vi "DequeueDependency.vi"(8 "error in (no error)":errorcluster, 11 "CDependencyQueue in":refnum<class "CDependencyQueue.lvclass">) -> (0 "error out":errorcluster, 1 "Shallow deps?":bool, 2 "Path":path, 3 "CDependencyQueue out":refnum<class "CDependencyQueue.lvclass">, 5 "timed out?":bool)   [LabVIEW 2020, in "DependencyInspection.lvlib" / "CDependencyQueue.lvclass"]
uses:
  CDependencyQueue.lvclass
  CDependencyQueue.lvclass/CDependencyQueue.ctl
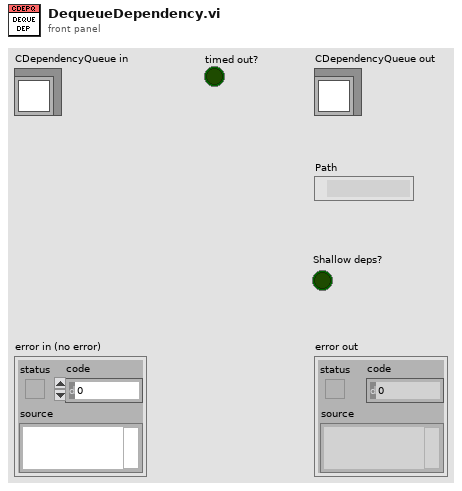
[diagram p1: front panel]
types:
  T1 = typedef "DependencyInspection.lvlib/CDependencyQueue.lvclass/DependencyQueue.ctl" = cluster{"New dependency":path, "Shallow dep?":bool}
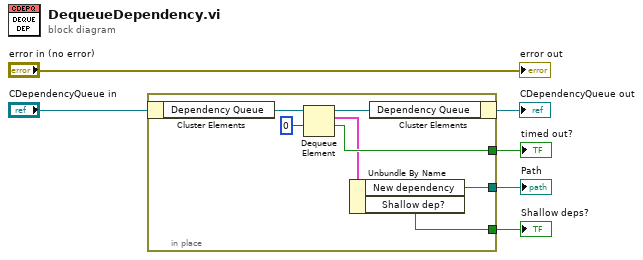
[diagram p0: block diagram]
diagram:
  n1 = in-place {
    in-place-border: [w9] -> w3
    in-place-border: [w7] -> w2
    in-place-border: [w6] -> w1
    n2 = in-place-cluster #1("CDependencyQueue in") -> ("Dependency Queue"=w11:refnum<queue>)
    n3 = Dequeue Element(queue=w11, timeout in ms (-1)=0) -> (queue out=w10:refnum<queue>, element=w8:T1, timed out?=w9:bool)  [unwired: 1 in, 1 out]
    n4 = Unbundle By Name(w8) -> ("New dependency"=w7:path, "Shallow dep?"=w6:bool)
    n5 = in-place-cluster #1("Dependency Queue"=w10) -> ()  [unwired: 1 out]
  }
  "timed out?" <- w3
  "Path" <- w2
  "Shallow deps?" <- w1
  "error out" <- "error in (no error)"
  "CDependencyQueue out" <- "CDependencyQueue in"
